vi "goToabsX.vi"(8 "error in":errorcluster, 11 "X position":dbl) -> (0 "error out":errorcluster)   [LabVIEW 2014]
doc: "André Romero - 2023\nandretec@ifsc.usp.br\nIFSC - USP"
uses:
  Global Motors.vi
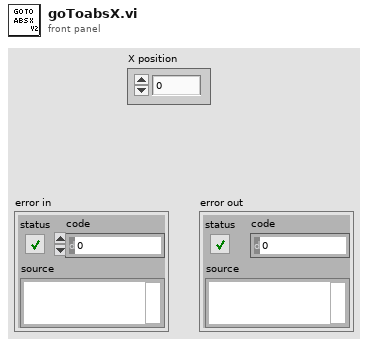
[diagram p1: front panel]
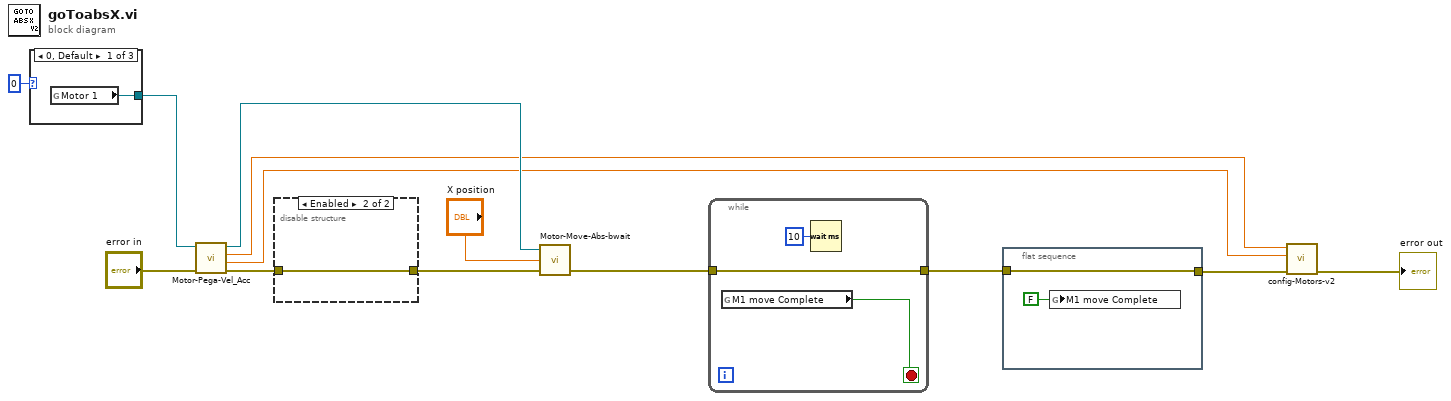
[diagram p0: block diagram]
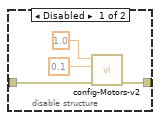
[diagram p2: hidden frame]
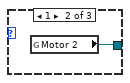
[diagram p3: hidden frame]
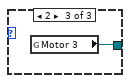
[diagram p4: hidden frame]
diagram:
  n1 = case shown="0, Default" u16 0 ("Axis") {
    tunnel: [w14 w15 w16] -> w6
    frame 0, Default {
      n2 = global read "Global Motors.vi" "Motor 1"() -> (w14:refnum<k7>)
    }
    frame 1 {
      n3 = global read "Global Motors.vi" "Motor 2"() -> (w15:refnum<k7>)
    }
    frame 2 {
      n4 = global read "Global Motors.vi" "Motor 3"() -> (w16:refnum<k7>)
    }
  }
  n5 = call "Motor-Pega-Vel_Acc.vi"("error out"="error in", "MG17Motor in"=w6) -> ("error out 2"=w9:errorcluster, "pfAccn"=w2:sgl, "pfMaxVel"=w1:sgl, "MG17Motor out"=w5:refnum<k7>)  [unwired: 2 in]
  n6 = disable-structure shown="Enabled" {
    disable-tunnel: w9 -> [w18 w21]
    disable-tunnel: [w17 w21] -> w8
    frame Disabled {
      n7 = call "config-Motors-v2.vi"("error in"=w18, "Acc"=0.1, "Velocity"=sgl 1.0) -> ("error out"=w17:errorcluster)  [unwired: 8 in]
    }
    frame Enabled {
    }
  }
  n8 = call "Motor-Move-Abs-bwait.vi"("error"=w8, "Posição"="X position", "MG17Motor A"=w5) -> ("error out"=w10:errorcluster)  [unwired: 1 in, 1 out]
  n9 = while {
    tunnel: w10 -> [w24]
    tunnel: [w24] -> w11
    stop <- w22 stop-if-true
    n10 = global read "Global Motors.vi" "M1 move Complete"() -> (w22:bool)
    n11 = Wait (ms)(milliseconds to wait=u32 10) -> ()  [unwired: 1 out]
  }
  n12 = flat-sequence {
    tunnel: w11 -> [w26]
    tunnel: [w26] -> w4
    frame #0 {
      n13 = global write "Global Motors.vi" "M1 move Complete"(FALSE ("M1 move Complete")) -> ()
    }
  }
  n14 = call "config-Motors-v2.vi"("error in"=w4, "Acc"=w2, "Velocity"=w1) -> ("error out"=→"error out":errorcluster)  [unwired: 8 in]
